vi "Create.vi"(8 "error in (no error)":errorcluster, 11 "Variant":variant) -> (0 "error out":errorcluster, 3 "Variant DVR out":refnum<data-value>)   [LabVIEW 2019, in "Variant Attributes.lvlib"]
doc: "Creates variant attribute DVR. You can set the value containted in the variant by wiring your data's wire to the input labelled as Variant."
uses:
  Variant Attributes.lvlib
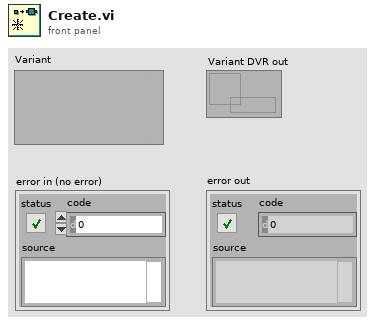
[diagram p1: front panel]
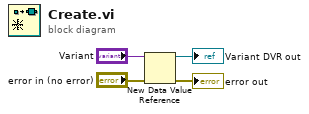
[diagram p0: block diagram]
diagram:
  n1 = New Data Value Reference(data value="Variant", error in="error in (no error)") -> (data value reference=→"Variant DVR out":refnum<data-value>, error out=→"error out":errorcluster)
